vi "LoopTime.vi"() -> (3 "LoopTime":u32)   [LabVIEW 2013]
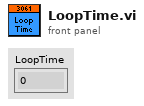
[diagram p1: front panel]
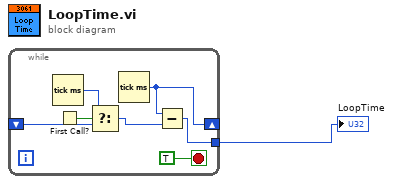
[diagram p0: block diagram]
diagram:
  n1 = while {
    shift-right: [w3] -> _
    shift-left: _ -> [w6]
    tunnel: [w2] -> w1
    stop <- TRUE stop-if-true
    n2 = Tick Count (ms)() -> (millisecond timer value=w5:u32)
    n3 = First Call?() -> (First Call?: T/F=w8:bool)
    n4 = Select(t=w5, s=w8, f=w6) -> (s? t:f=w7:u32)
    n5 = Tick Count (ms)() -> (millisecond timer value=w3:u32)
    n6 = Subtract(x=w3, y=w7) -> (x-y=w2:u32)
  }
  "LoopTime" <- w1
